vi "Interpolate Y.vi"   [LabVIEW 2019, in "xy_utilities.lvlib"]
doc: "Given a fractional x value, interpolate a factional y value.\n\nWire data to the data input to determine the polymorphic instance to use or manually select the instance."
uses:
  xy_utilities.lvlib
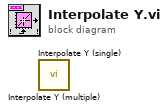
[diagram p0: block diagram]
diagram:
  n1 = call "Interpolate Y (multiple).vi"() -> ()  [unwired: 9 in, 3 out]
  n2 = call "Interpolate Y (single).vi"() -> ()  [unwired: 9 in, 3 out]
